vi "Compute DistanceToTarget2.vi"(9 "Camera Type":T3, 10 "Line":T1, 11 "Image Src":T2) -> (2 "Distance (ft)":dbl, 3 "Image Dst Out":T2)   [LabVIEW 2023]
doc: "Using the camera lens information and the real world size of the target, use trig and ratios to determine the distance to the target. Also returns the location relative to the image center in a (-1 , 1) coordinate system that may be useful for steering the robot."
uses:
  Camera Types.ctl
  <vilib>/vision/Image Controls.llb/IMAQ Image.ctl
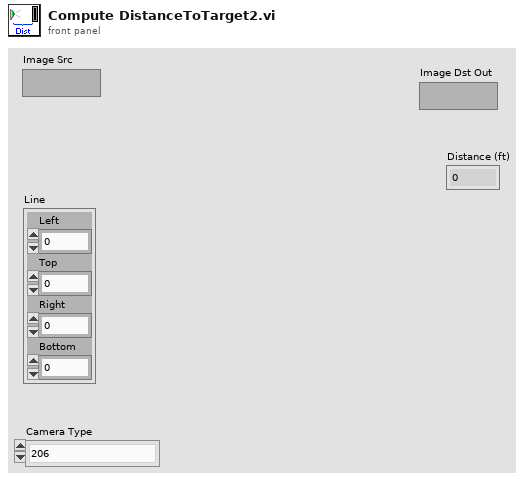
[diagram p1: front panel]
types:
  T1 = cluster{"Left":dbl, "Top":dbl, "Right":dbl, "Bottom":dbl}
  T2 = typedef "IMAQ Image.ctl" = refnum<image>
  T3 = typedef "Camera Types.ctl" = enum16{"206", "1011", "1013", "MS HD3000 square", "MS HD3000 640x480", "MS HD3000 1280x720"}
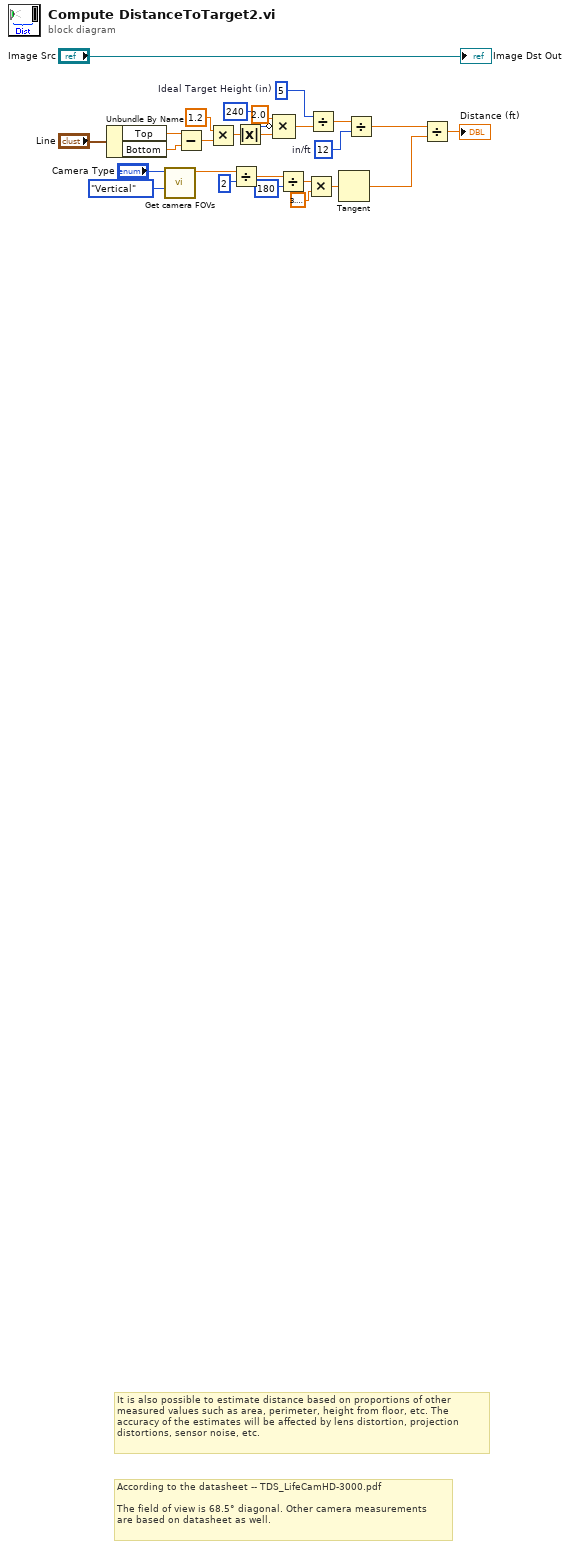
[diagram p0: block diagram]
diagram:
  w13 = 5  # Ideal Target Height (in)
  w20 = 12  # in/ft
  # "It is also possible to estimate distance based on proportions of other\nmeasured values such as area, perimeter, height from floor, etc. The\naccuracy of the estimates will be affected by lens distortion, projection\ndistortions, sensor noise, etc."
  # "According to the datasheet -- TDS_LifeCamHD-3000.pdf\n\nThe field of view is 68.5° diagonal. Other camera measurements\nare based on datasheet as well."
  n1 = Unbundle By Name("Line") -> ("Top"=w8:dbl, "Bottom"=w7:dbl)
  n2 = call "Get camera FOVs.vi"("Type"=enum16{"Horizontal", "Vertical", "Diagonal"}."Vertical" ("Angle"), "Camera Type"="Camera Type") -> ("FOV"=w15:dbl)  [unwired: 8 in, 1 out]
  n3 = Subtract(x=w8, y=w7) -> (x-y=w5:dbl)
  n4 = Multiply(x=1.2, y=w5) -> (x*y=w4:dbl)
  n5 = Divide(x=w15, y=2) -> (x/y=w23:dbl)
  n6 = Absolute Value(x=w4) -> (abs(x)=w6:dbl)
  n7 = Compound Arithmetic op=MULTIPLY(2.0, invert 240 ("Y Resolution"), w6) -> (w11:dbl)
  n8 = Divide(x=w23, y=180) -> (x/y=w22:dbl)
  n9 = Multiply(x=w22, y=3.141592653589793) -> (x*y=w24:dbl)
  n10 = Divide(x=w13, y=w11) -> (x/y=w17:dbl)
  n11 = Tangent(1:w24) -> (0:w19:dbl)
  n12 = Divide(x=w17, y=w20) -> (x/y=w16:dbl)
  n13 = Divide(x=w16, y=w19) -> (x/y=→"Distance (ft)":dbl)
  "Image Dst Out" <- "Image Src"
